vi "Transmit Datagram.vi"(5 "transfer id":i32, 7 "transfer group id":i32, 8 "error in (no error)":errorcluster, 9 "transfer data":string, 11 "UDP Transceiver in":refnum<class "UDP Transceiver.lvclass">) -> (0 "error out":errorcluster, 1 "timed out?":bool, 3 "UDP Transceiver out":refnum<class "UDP Transceiver.lvclass">)   [LabVIEW 2020, in "UDP.lvlib" / "UDP Transceiver.lvclass"]
uses:
  UDP Transceiver.lvclass
  UDP Transceiver.lvclass/UDP Transceiver.ctl
  <vilib>/Utility/error.llb/Clear Errors.vi
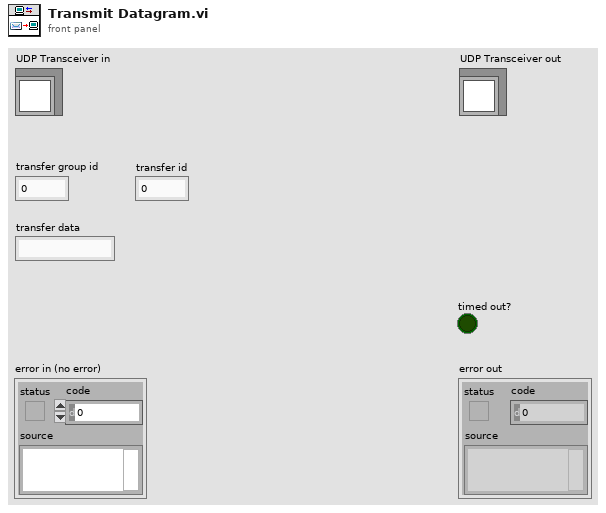
[diagram p1: front panel]
types:
  T1 = typedef "UDP.lvlib/UDP Transceiver.lvclass/Transfer Group Parameters.ctl" = cluster{"transfers":T2[], "max size":i32, "timeout":i32}
  T2 = typedef "UDP.lvlib/UDP Transceiver.lvclass/Transfer Parameters.ctl" = cluster{"group offset":u64, "size":u64, "address":u32, "port":u16}
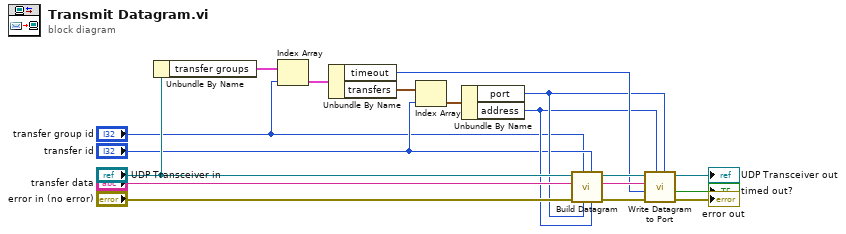
[diagram p0: block diagram]
diagram:
  n1 = Unbundle By Name("UDP Transceiver in") -> ("transfer groups"=w10:T1[])
  n2 = Index Array(array=w10, index="transfer group id") -> (element=w9:T1)
  n3 = Unbundle By Name(w9) -> ("timeout"=w6:i32, "transfers"=w7:T2[])
  n4 = Index Array(array=w7, index="transfer id") -> (element=w8:T2)
  n5 = Unbundle By Name(w8) -> ("port"=w5:u16, "address"=w4:u32)
  n6 = call-dynamic "Build Datagram.vi"("destination address"=w4, "transfer id"="transfer id", "destination port"=w5, "transfer group id"="transfer group id", "error in (no error)"="error in (no error)", "transfer data"="transfer data", "UDP Transceiver in"="UDP Transceiver in") -> ("error out"=w14:errorcluster, "datagram"=w15:string, "UDP Transceiver out"=w11:refnum<class "UDP Transceiver.lvclass">)  [unwired: 2 in]
  n7 = call "Write Datagram to Port.vi"("destination port"=w5, "destination address"=w4, "error in (no error)"=w14, "timeout ms (25000)"=w6, "data"=w15, "UDP Transceiver in"=w11) -> ("error out"=→"error out":errorcluster, "timed out?"=→"timed out?":bool, "UDP Transceiver out"=→"UDP Transceiver out":refnum<class "UDP Transceiver.lvclass">)  [unwired: 3 in]
